vi "Ramp.vi"(1 "initial output (%)":dbl format="%.2f", 2 "run (T)":bool=TRUE, 3 "initialize":bool, 4 "cycle time (sec)":dbl=1.0 format="%.2f", 5 "rate (%/min)":dbl format="%.2f", 6 "setpoint (%)":dbl format="%.2f") -> (0 "output (%)":dbl format="%.4f")   [LabVIEW 2020, in "NI_PID__prctrl compat.lvlib"]
doc: "Setpoint ramp generator. Output ramps linearly toward the setpoint at \"Rate\" percent per minute. Sign (+ or -) of Rate determines polarity of ramp.\n\nSetpoint and output are expressed in percent. Output can be forced to a desired value by setting Initialize to TRUE. \"Initial Value\" is then written into the output. Setting \"Run\" to FALSE makes the output hold at the last value. Initialize overrides Run.\n\nThis VI should be called from inside a while loop with a fixed cycle time. Note that the cycle time (part of the Tuning Parameters) is in seconds and MUST be supplied; control calibration depends on this value. This VI is reentrant, so you can call it from multiple, independent higher-level VIs without interference."
uses:
  <vilib>/addons/control/pid/NI_PID__prctrl compat.lvlib
panel:
  # "Ramp Generator"
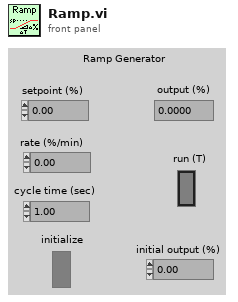
[diagram p1: front panel]
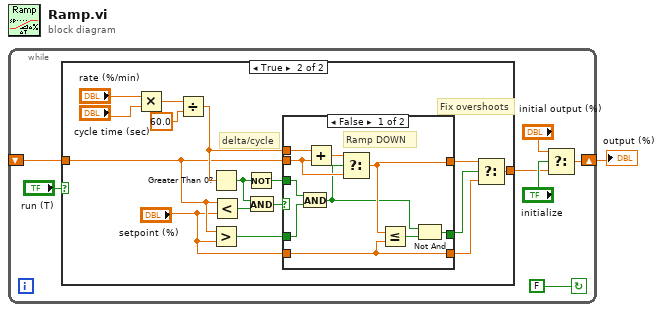
[diagram p0: block diagram]
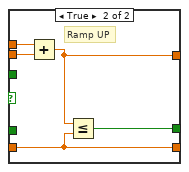
[diagram p3: hidden frame]
diagram:
  n1 = while {
    shift-left: _ -> [w4]
    shift-right: [w6] -> w1
    stop <- FALSE continue-if-true
    n2 = case shown="True" "run (T)" {
      tunnel: [w9 w13] -> w3
      tunnel: w4 -> [w9 w17]
      frame False {
      }
      frame True {
        # "Fix overshoots"
        # "delta/cycle"
        n3 = Multiply(x="rate (%/min)", y="cycle time (sec)") -> (x*y=w23:dbl)
        n4 = Divide(x=w23, y=60.0) -> (x/y=w21:dbl)
        n5 = Greater Than 0?(x=w21) -> (x > 0?=w19:bool)
        n6 = Greater?(x=w17, y="setpoint (%)") -> (0:w16:bool)
        n7 = Less?(x=w17, y="setpoint (%)") -> (x < y?=w20:bool)
        n8 = Not(x=w19) -> (.not. x?=w18:bool)
        n9 = And(x=w19, y=w20) -> (x .and. y?=w22:bool)
        n10 = case shown="False" w22 {
          tunnel: [w31 w36] -> w11
          tunnel: [w27 w37] -> w14
          tunnel: "setpoint (%)" -> [w31 w36]
          tunnel: w18 -> [w34 _]
          tunnel: w16 -> [w35 _]
          tunnel: [w29 w38] -> w12
          tunnel: w21 -> [w33 w39]
          tunnel: w17 -> [w32 w40]
          frame False {
            # "Ramp DOWN"
            n11 = And(x=w34, y=w35) -> (x .and. y?=w26:bool)
            n12 = Add(x=w33, y=w32) -> (x+y=w30:dbl)
            n13 = Select(t=w30, s=w26, f=w32) -> (s? t:f=w29:dbl)
            n14 = Less Or Equal?(x=w29, y=w31) -> (x <= y?=w28:bool)
            n15 = Not And(1:w28, 2:w26) -> (0:w27:bool)
          }
          frame True {
            # "Ramp UP"
            n16 = Add(x=w39, y=w40) -> (x+y=w38:dbl)
            n17 = Less Or Equal?(x=w38, y=w36) -> (x <= y?=w37:bool)
          }
        }
        n18 = Select(t=w12, s=w14, f=w11) -> (s? t:f=w13:dbl)
      }
    }
    n19 = Select(t="initial output (%)", s="initialize", f=w3) -> (s? t:f=w6:dbl)
  }
  "output (%)" <- w1
